vi "Write listaDePruebas.vi"(8 "error in (no error)":errorcluster, 10 "listaDePruebas":refnum<class "Prueba.lvclass">[](array[class]), 11 "Dosimetro in":refnum<class "Dosimetro.lvclass">) -> (0 "error out":errorcluster, 3 "Dosimetro out":refnum<class "Dosimetro.lvclass">)   [LabVIEW 2019, in "Dosimetro.lvclass"]
uses:
  Dosimetro.lvclass
  Pruebas/Prueba/Prueba.lvclass
  Dosimetro.lvclass/Dosimetro.ctl
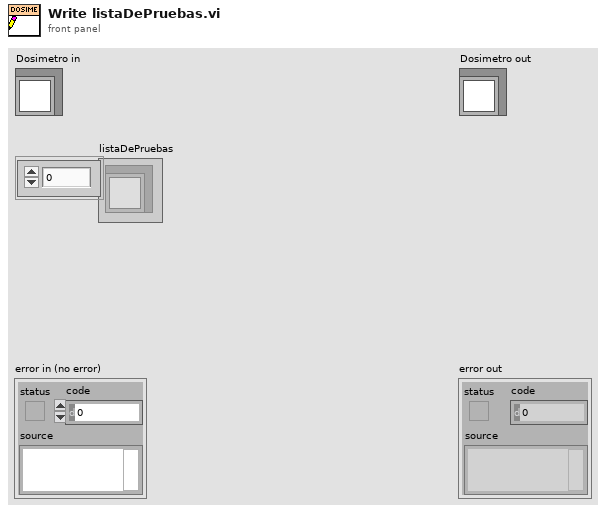
[diagram p1: front panel]
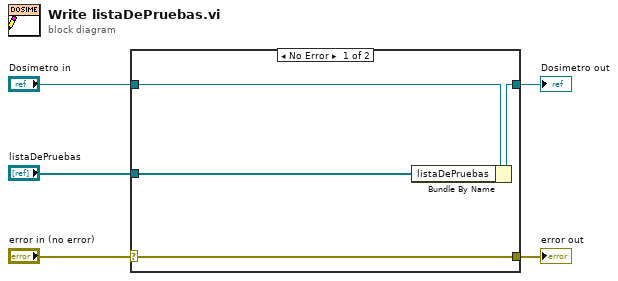
[diagram p0: block diagram]
diagram:
  n1 = case shown="No Error" "error in (no error)" {
    selector: "error in (no error)" -> [w9 w10]
    tunnel: [w9 w10] -> w4
    tunnel: [w7 w11] -> w2
    tunnel: "Dosimetro in" -> [w8 w11]
    tunnel: "listaDePruebas" -> [w6 _]
    frame No Error {
      n2 = Bundle By Name(cluster=w8, "listaDePruebas"=w6) -> (w7:refnum<class "Dosimetro.lvclass">)
    }
    frame Error {
    }
  }
  "error out" <- w4
  "Dosimetro out" <- w2
